vi "RSZVB Get Marker Search Range Show.vi"(8 "error in (no error)":errorcluster {"code" format="%.0x"}, 9 "Marker (1)":i32=1, 10 "Channel (Trace) (1)":i32=1, 11 "VISA session":refnum<visa-resource-name>) -> (0 "error out":errorcluster {"code" format="%.0x"}, 3 "dup VISA session":refnum<visa-resource-name>, 7 "Show Range (F: Off)":bool)   [LabVIEW 2011]
doc: "Queries whether range limit lines for the search range are displayed.\n\nRemote-control command(s):\nCALCulate<Chn>:MARKer<Mk>:FUNCtion:DOMain:USER:SHOW?"
panel:
  # "On\nOff"
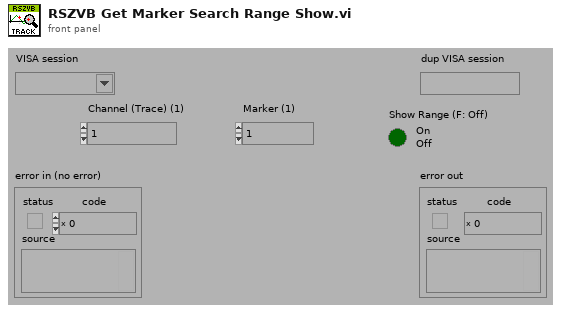
[diagram p1: front panel]
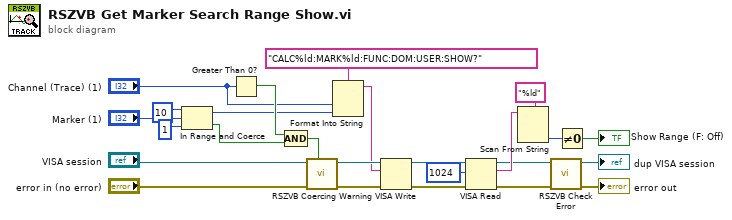
[diagram p0: block diagram]
diagram:
  n1 = In Range and Coerce(upper limit=10, x="Marker (1)", lower limit=1) -> (coerced(x)=w17:i32, In Range?=w10:bool)
  n2 = Greater Than 0?(x="Channel (Trace) (1)") -> (x > 0?=w20:bool)
  n3 = Compound Arithmetic op=AND(w20, w10) -> (w22:bool)
  n4 = call "RSZVB Coercing Warning.vi"("In Range?"=w22, "error in (no error)"="error in (no error)", "VISA session"="VISA session") -> ("error out"=w23:errorcluster, "dup VISA session"=w24:refnum<visa-resource-name>)  [unwired: 7 in]
  n5 = Format Into String(format string="CALC%ld:MARK%ld:FUNC:DOM:USER:SHOW?", "Channel (Trace) (1)", w17) -> (resulting string=w21:string)  [unwired: 2 in, 1 out]
  n6 = VISA Write(VISA resource name=w24, write buffer=w21, error in (no error)=w23) -> (VISA resource name out=w6:refnum<visa-resource-name>, error out=w5:errorcluster)  [unwired: 1 out]
  n7 = VISA Read(VISA resource name=w6, byte count=u32 1024 ("byte count (0)"), error in (no error)=w5) -> (VISA resource name out=w2:refnum<visa-resource-name>, read buffer=w3:string, error out=w1:errorcluster)  [unwired: 1 out]
  n8 = Scan From String(format string="%ld", input string=w3) -> (output 1=w7:i32)  [unwired: 3 in, 3 out]
  n9 = call "RSZVB Check Error.vi"("error in (no error)"=w1, "VISA session"=w2) -> ("error out"=→"error out":errorcluster, "dup VISA session"=→"dup VISA session":refnum<visa-resource-name>)  [unwired: 8 in]
  n10 = Not Equal To 0?(x=w7) -> (x != 0?=→"Show Range (F: Off)":bool)
